vi "WSVCAP SHL Host LL Set Read_Write Parameters.vi"(0 "Transaction":T1, 1 "Wait Ticks":u32, 2 "Slave Address":u8, 5 "Bytes":u8, 7 "Sub Address [U8]":u8=191 format="%.0x", 9 "Socket Mask [U64]":u64=1 format="%016x", 11 "error in (no error)":errorcluster, 12 "UUT Set (0/1)":u8) -> (15 "error out":errorcluster)   [LabVIEW 2012]
uses:
  Type Defs/WSVCAP SHL Transaction Enum.ctl
  Type Defs/WSVCAP SHL Top Level Control Operation Enum.ctl
  Type Defs/WSVCAP SHL State.ctl
  Type Defs/WSVCAP SHL Top Level Control Enum.ctl
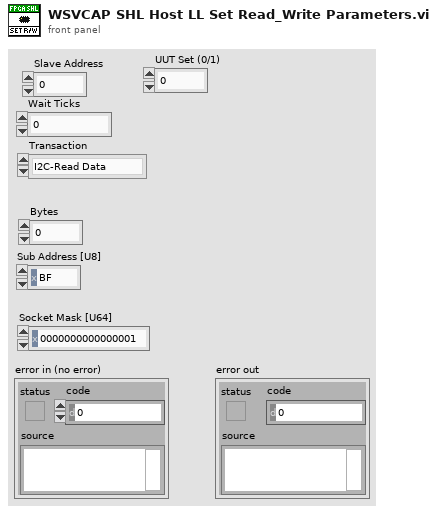
[diagram p1: front panel]
types:
  T1 = typedef "WSVCAP SHL Transaction Enum.ctl" = enum16{"I2C-Read Data", "I2C-Write Data", "RFFE-Ext Write", "RFFE-Ext Read"}
  T2 = typedef "WSVCAP SHL Top Level Control Enum.ctl" = enum16{"Start", "Cmd", "Transaction", "Wait Ticks", "Socket Mask", "UUT Set", "Slave Address", "Sub Address", "Bytes to Write", "Bytes to Read", "Write Data", "Write Flag", "Read Data", "Read Flag", "Ack Read", "Read Status Flag", "Ack Read Status", "Status", "Cycle Count", "Stop Cycle", "Exit"}
  T3 = typedef "WSVCAP SHL State.ctl" = enum8{"Idle", "Transfer Data"}
  T4 = typedef "WSVCAP SHL Top Level Control Operation Enum.ctl" = enum16{"Initialize", "Set Control", "Read Control", "Close"}
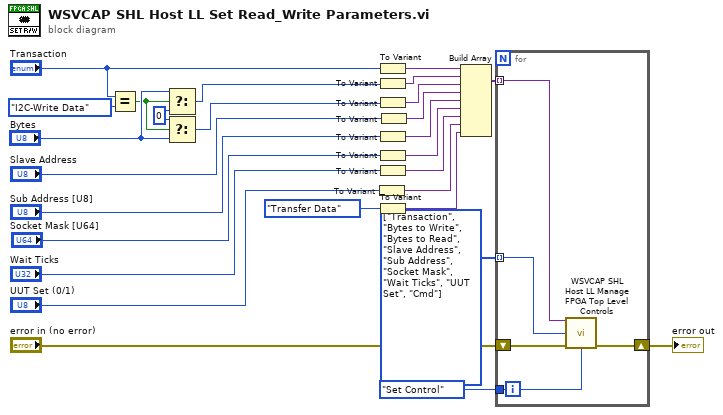
[diagram p0: block diagram]
diagram:
  w18 = u8 0 ("t")
  w20 = T2[] [enum."Transaction", enum."Bytes to Write", enum."Bytes to Read", enum."Slave Address", enum."Sub Address", enum."Socket Mask", enum."Wait Ticks", enum."UUT Set", enum."Cmd"] items=["Start", "Cmd", "Transaction", "Wait Ticks", "Socket Mask", "UUT Set", "Slave Address", "Sub Address", "Bytes to Write", "Bytes to Read", "Write Data", "Write Flag", "Read Data", "Read Flag", "Ack Read", "Read Status Flag", "Ack Read Status", "Status", "Cycle Count", "Stop Cycle", "Exit"]
  n1 = Equal?(x="Transaction", y=WSVCAP_SHL_Transaction_Enum."I2C-Write Data" ("Transaction")) -> (x = y?=w12:bool)
  n2 = Select(t="Bytes", s=w12, f=w18) -> (s? t:f=w17:u8)
  n3 = Select(t=w18, s=w12, f="Bytes") -> (s? t:f=w16:u8)
  n4 = To Variant(anything="UUT Set (0/1)") -> (Variant=w1:variant)
  n5 = To Variant(anything="Transaction") -> (Variant=w26:variant)
  n6 = To Variant(anything=w17) -> (Variant=w25:variant)
  n7 = To Variant(anything=w16) -> (Variant=w15:variant)
  n8 = To Variant(anything="Sub Address [U8]") -> (Variant=w11:variant)
  n9 = To Variant(anything="Socket Mask [U64]") -> (Variant=w10:variant)
  n10 = To Variant(anything="Wait Ticks") -> (Variant=w6:variant)
  n11 = To Variant(anything=WSVCAP_SHL_State."Transfer Data" ("SPI_Cmd")) -> (Variant=w21:variant)
  n12 = To Variant(anything="Slave Address") -> (Variant=w3:variant)
  n13 = Build Array(w26, w25, w15, w3, w11, w10, w6, w1, w21) -> (w24:variant[])
  n14 = for {
    tunnel: WSVCAP_SHL_Top_Level_Control_Operation_Enum."Set Control" ("Operation") -> [w32]
    tunnel: w24 -> [w31] mode=indexing
    tunnel: w20 -> [w30] mode=indexing
    shift-right: [w28] -> w22
    shift-left: "error in (no error)" -> [w29]
    n15 = call "WSVCAP SHL Host LL Manage FPGA Top Level Controls.vi"("Value In"=w31, "FPGA Top Level Control"=w30, "error in (no error)"=w29, "Operation"=w32) -> ("error out"=w28:errorcluster)  [unwired: 10 in, 1 out]
  }
  "error out" <- w22
